vi "task1.vi"() -> ()   [LabVIEW 2017]
panel:
  in  "Boolean 16":bool
  in  "Boolean 15":bool
  in  "Boolean 14":bool
  in  "Boolean 13":bool
  in  "Boolean 12":bool
  in  "Boolean 11":bool
  in  "Boolean 10":bool
  out "Boolean 9":bool
  out "Boolean 8":bool
  out "Boolean 7":bool
  out "Boolean 6":bool
  out "Boolean 5":bool
  out "Boolean 4":bool
  in  "Boolean 3":bool
  out "Boolean 2":bool
  out "Boolean":bool
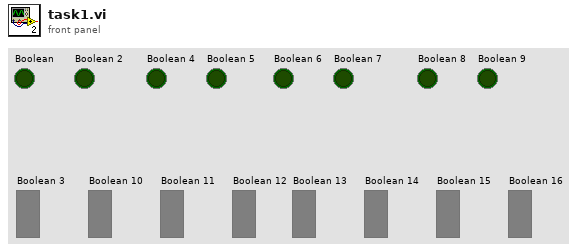
[diagram p1: front panel]
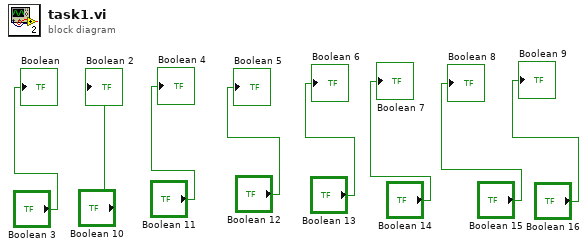
[diagram p0: block diagram]
diagram:
  "Boolean" <- "Boolean 3"
  "Boolean 2" <- "Boolean 10"
  "Boolean 4" <- "Boolean 11"
  "Boolean 5" <- "Boolean 12"
  "Boolean 6" <- "Boolean 13"
  "Boolean 7" <- "Boolean 14"
  "Boolean 8" <- "Boolean 15"
  "Boolean 9" <- "Boolean 16"
